vi "Variant Tools Test.vi"() -> ()   [LabVIEW 2017]
uses:
  c802287c-51b3-4527-ae67-bf64e1a5bd7d.vi
  fdbdbf5d-b64d-4e2e-bc22-f5c9394cad9c.vi
  <vilib>/addons/JSON API/JSON Value/Set from JSON string.vi
  Variant to JSON Text.vi
  JSON text to Variant.vi
  <vilib>/addons/JSON API/Variant JSON/Get as Variant.vi
  <vilib>/addons/JSON API/JSON Value/JSON Value.lvclass
  <vilib>/gmath/NI_Gmath.lvlib
  <vilib>/addons/JSON API/Get Polymorphic/JSON GetSet.lvlib
  <vilib>/addons/JSON API/Variant JSON/Variant JSON.lvlib
panel:
  in  "Pretty Print?":bool=TRUE
  out "x = y? 2":T1
  out "Cluster 2":T2={"A 6"=34, "T 1"="L", "A"=3, "<JSON>T 3"="", "T 4"="", "A 2"=1.23456, "T 5"="Test \"quote\",\nand newline.", "T 6"="sdfsdf", "A 3"=34, "Cluster 2"={"T 1"="SubCluster", "T 2"="Test \"quote\",\nand newline.", "A"=34, "T 3"="Test \"quote\",\nand newline.", "T 4"="Test \"quote\",\nand newline.", "A 2"=34, "T 5"="Test \"quote\",\nand newline.", "T 6"="Test \"quote\",\nand newline.", "A 3"=34}, "Array"=[1.23456, 1.23456, 1.23456, 1.23456, 1.23456, 1.23456, 1.23456, 1.23456, 1.23456, 1.23456, 1.23456, 1.23456, 2.23456]}
  in  "Old JSON":bool
  out "mean":dbl format="%.3p"
  out "length":i32
  out "Variant out":variant
  out "To Variant":dbl[](array[numeric]) format="%#_3p"
  in  "Cluster":T2={"A 6"=34, "T 1"="Line 1", "A"=34, "<JSON>T 3"="{\"T\":123}", "T 4"="sdfsdfdsfsdf", "A 2"=1.23456, "T 5"="Test \"quote\",\nand newline.", "T 6"="sdfsdf", "A 3"=34, "Cluster 2"={"T 1"="SubCluster", "T 2"="Test \"quote\",\nand newline.", "A"=34, "T 3"="Test \"quote\",\nand newline.", "T 4"="Test \"quote\",\nand newline.", "A 2"=34, "T 5"="Test \"quote\",\nand newline.", "T 6"="Test \"quote\",\nand newline.", "A 3"=34}, "Array"=[1.23456789, 1.23456789, 1.23456789, 1.23456789, 1.23456789, 1.23456789, 1.23456789, 1.23456789, 1.23456789, 1.23456789, 1.23456789, 1.23456789, 1.23456789, 1.23456789, 1.23456789, 1.23456789, 1.23456789, 1.23456789, 1.23456789, 1.23456789, 1.23456789, 1.23456789, 1.23456789, 1.23456789, 1.23456789, 1.23456789, 1.23456789, 1.23456789, 1.23456789, 1.23456789, 1.23456789, 1.23456789, 1.23456789, 1.23456789, 1.23456789, 1.23456789, 1.23456789, 1.23456789, 1.23456789, 1.23456789, 1.23456789, 1.23456789, 1.23456789, 1.23456789, 1.23456789, 1.23456789, 1.23456789, 1.23456789, 1.23456789, 1.23456789, 1.23456789, 1.23456789, 1.23456789, 1.23456789, 1.23456789, 1.23456789, 1.23456789, 1.23456789, 1.23456789, 1.23456789, 1.23456789, 1.23456789, 1.23456789, 1.23456789, 1.23456789, 1.23456789, 1.23456789, 1.23456789, 1.23456789, 1.23456789, 1.23456789, 1.23456789, 1.23456789, 1.23456789, 1.23456789, 1.23456789, 1.23456789, 1.23456789, 1.23456789, 1.23456789, 1.23456789, 1.23456789, 1.23456789, 1.23456789, 1.23456789, 1.23456789, 1.23456789, 1.23456789, 1.23456789, 1.23456789, 1.23456789, 1.23456789, 1.23456789, 1.23456789, 1.23456789, 1.23456789, 1.23456789, 1.23456789, 1.23456789, 1.23456789, 1.23456789, 1.23456789, 1.23456789, 1.23456789, 1.23456789, 1.23456789, 1.23456789, 1.23456789, 1.23456789, 1.23456789, 1.23456789, 1.23456789, 1.23456789, 1.23456789, 1.23456789, 1.23456789, 1.23456789, 1.23456789, 1.23456789, 1.23456789, 1.23456789, 1.23456789, 1.23456789, 1.23456789, 1.23456789, 1.23456789, 1.23456789, 1.23456789, 1.23456789, 1.23456789, 1.23456789, 1.23456789, 1.23456789, 1.23456789, 1.23456789, 1.23456789, 1.23456789, 1.23456789, 1.23456789, 1.23456789, 1.23456789, 1.23456789, 1.23456789, 1.23456789, 1.23456789, 1.23456789, 1.23456789, 1.23456789, 1.23456789, 1.23456789, 1.23456789, 1.23456789, 1.23456789, 1.23456789, 1.23456789, 1.23456789, 1.23456789, 1.23456789, 1.23456789, 1.23456789, 1.23456789, 1.23456789, 1.23456789, 1.23456789, 1.23456789, 1.23456789, 1.23456789, 1.23456789, 1.23456789, 1.23456789, 1.23456789, 1.23456789, 1.23456789, 1.23456789, 1.23456789, 1.23456789, 1.23456789, 1.23456789, 1.23456789, 1.23456789, 1.23456789, 1.23456789, 1.23456789, 1.23456789, 1.23456789, 1.23456789, 1.23456789, 1.23456789, 1.23456789, 1.23456789, 1.23456789, 1.23456789, 1.23456789, 1.23456789, 1.23456789, 1.23456789, 1.23456789, 1.23456789, 1.23456789, 1.23456789, 1.23456789, 1.23456789, 1.23456789, 1.23456789, 1.23456789, 1.23456789, 1.23456789, 1.23456789, 1.23456789, 1.23456789, 1.23456789, 1.23456789, 1.23456789, 1.23456789, 1.23456789, 1.23456789, 1.23456789, 1.23456789, 1.23456789, 1.23456789, 1.23456789, 1.23456789, 1.23456789, 1.23456789, 1.23456789, 1.23456789, 1.23456789, 1.23456789, 1.23456789, 1.23456789, 1.23456789, 1.23456789, 1.23456789, 1.23456789, 1.23456789, 1.23456789, 1.23456789, 1.23456789, 1.23456789, 1.23456789, 1.23456789, 1.23456789, 1.23456789, 1.23456789, 1.23456789, 1.23456789, 1.23456789, 1.23456789, 1.23456789, 1.23456789, 1.23456789, 1.23456789, 1.23456789, 1.23456789, 1.23456789, 1.23456789, 1.23456789, 1.23456789, 1.23456789, 1.23456789, 1.23456789, 1.23456789, 1.23456789, 1.23456789, 1.23456789, 1.23456789, 1.23456789, 1.23456789, 1.23456789, 1.23456789, 1.23456789, 1.23456789, 1.23456789, 1.23456789, 1.23456789, 1.23456789, 1.23456789, 1.23456789, 1.23456789, 1.23456789, 1.23456789, 1.23456789, 1.23456789, 1.23456789, 1.23456789, 1.23456789, 1.23456789, 1.23456789, 1.23456789, 1.23456789, 1.23456789, 1.23456789, 1.23456789, 1.23456789, 1.23456789, 1.23456789, 1.23456789, 1.23456789, 1.23456789, 1.23456789, 1.23456789, 1.23456789, 1.23456789, 1.23456789, 1.23456789, 1.23456789, 1.23456789, 1.23456789, 1.23456789, 1.23456789, 1.23456789, 1.23456789, 1.23456789, 1.23456789, 1.23456789, 1.23456789, 1.23456789, 1.23456789, 1.23456789, 1.23456789, 1.23456789, 1.23456789, 1.23456789, 1.23456789, 1.23456789, 1.23456789, 1.23456789, 1.23456789, 1.23456789, 1.23456789, 1.23456789, 1.23456789, 1.23456789, 1.23456789, 1.23456789, 1.23456789, 1.23456789, 1.23456789, 1.23456789, 1.23456789, 1.23456789, 1.23456789, 1.23456789, 1.23456789, 1.23456789, 1.23456789, 1.23456789, 1.23456789, 1.23456789, 1.23456789, 1.23456789, 1.23456789, 1.23456789, 1.23456789, 1.23456789, 1.23456789, 1.23456789, 1.23456789, 1.23456789, 1.23456789, 1.23456789, 1.23456789, 1.23456789, 1.23456789, 1.23456789, 1.23456789, 1.23456789, 1.23456789, 1.23456789, 1.23456789, 1.23456789, 1.23456789, 1.23456789, 1.23456789, 1.23456789, 1.23456789, 1.23456789, 1.23456789, 1.23456789, 1.23456789, 1.23456789, 1.23456789, 1.23456789, 1.23456789, 1.23456789, 1.23456789, 1.23456789, 1.23456789, 1.23456789, 1.23456789, 1.23456789, 1.23456789, 1.23456789, 1.23456789, 1.23456789, 1.23456789, 1.23456789, 1.23456789, 1.23456789, 1.23456789, 1.23456789, 1.23456789, 1.23456789, 1.23456789, 1.23456789, 1.23456789, 1.23456789, 1.23456789, 1.23456789, 1.23456789, 1.23456789, 1.23456789, 1.23456789, 1.23456789, 1.23456789, 1.23456789, 1.23456789, 1.23456789, 1.23456789, 1.23456789, 1.23456789, 1.23456789, 1.23456789, 1.23456789, 1.23456789, 1.23456789, 1.23456789, 1.23456789, 1.23456789, 1.23456789, 1.23456789, 1.23456789, 1.23456789, 1.23456789, 1.23456789, 1.23456789, 1.23456789, 1.23456789, 1.23456789, 1.23456789, 1.23456789, 1.23456789, 1.23456789, 1.23456789, 1.23456789, 1.23456789, 1.23456789, 1.23456789, 1.23456789, 1.23456789, 1.23456789, 1.23456789, 1.23456789, 1.23456789, 1.23456789, 1.23456789, 1.23456789, 1.23456789, 1.23456789, 1.23456789, 1.23456789, 1.23456789, 1.23456789, 1.23456789, 1.23456789, 1.23456789, 1.23456789, 1.23456789, 1.23456789, 1.23456789, 1.23456789, 1.23456789, 1.23456789, 1.23456789, 1.23456789, 1.23456789, 1.23456789, 1.23456789, 1.23456789, 1.23456789, 1.23456789, 1.23456789, 1.23456789, 1.23456789, 1.23456789, 1.23456789, 1.23456789, 1.23456789, 1.23456789, 1.23456789, 1.23456789, 1.23456789, 1.23456789, 1.23456789, 1.23456789, 1.23456789, 1.23456789, 1.23456789, 1.23456789, 1.23456789, 1.23456789, 1.23456789, 1.23456789, 1.23456789, 1.23456789, 1.23456789, 1.23456789, 1.23456789, 1.23456789, 1.23456789, 1.23456789, 1.23456789, 1.23456789, 1.23456789, 1.23456789, 1.23456789, 1.23456789, 1.23456789, 1.23456789, 1.23456789, 1.23456789, 1.23456789, 1.23456789, 1.23456789, 1.23456789, 1.23456789, 1.23456789, 1.23456789, 1.23456789, 1.23456789, 1.23456789, 1.23456789, 1.23456789, 1.23456789, 1.23456789, 1.23456789, 1.23456789, 1.23456789, 1.23456789, 1.23456789, 1.23456789, 1.23456789, 1.23456789, 1.23456789, 1.23456789, 1.23456789, 1.23456789, 1.23456789, 1.23456789, 1.23456789, 1.23456789, 1.23456789, 1.23456789, 1.23456789, 1.23456789, 1.23456789, 1.23456789, 1.23456789, 1.23456789, 1.23456789, 1.23456789, 1.23456789, 1.23456789, 1.23456789, 1.23456789, 1.23456789, 1.23456789, 1.23456789, 1.23456789, 1.23456789, 1.23456789, 1.23456789, 1.23456789, 1.23456789, 1.23456789, 1.23456789, 1.23456789, 1.23456789, 1.23456789, 1.23456789, 1.23456789, 1.23456789, 1.23456789, 1.23456789, 1.23456789, 1.23456789, 1.23456789, 1.23456789, 1.23456789, 1.23456789, 1.23456789, 1.23456789, 1.23456789, 1.23456789, 1.23456789, 1.23456789, 1.23456789, 1.23456789, 1.23456789, 1.23456789, 1.23456789, 1.23456789, 1.23456789, 1.23456789, 1.23456789, 1.23456789, 1.23456789, 1.23456789, 1.23456789, 1.23456789, 1.23456789, 1.23456789, 1.23456789, 1.23456789, 1.23456789, 1.23456789, 1.23456789, 1.23456789, 1.23456789, 1.23456789, 1.23456789, 1.23456789, 1.23456789, 1.23456789, 1.23456789, 1.23456789, 1.23456789, 1.23456789, 1.23456789, 1.23456789, 1.23456789, 1.23456789, 1.23456789, 1.23456789, 1.23456789, 1.23456789, 1.23456789, 1.23456789, 1.23456789, 1.23456789, 1.23456789, 1.23456789, 1.23456789, 1.23456789, 1.23456789, 1.23456789, 1.23456789, 1.23456789, 1.23456789, 1.23456789, 1.23456789, 1.23456789, 1.23456789, 1.23456789, 1.23456789, 1.23456789, 1.23456789, 1.23456789, 1.23456789, 1.23456789, 1.23456789, 1.23456789, 1.23456789, 1.23456789, 1.23456789, 1.23456789, 1.23456789, 1.23456789, 1.23456789, 1.23456789, 1.23456789, 1.23456789, 1.23456789, 1.23456789, 1.23456789, 1.23456789, 1.23456789, 1.23456789, 1.23456789, 1.23456789, 1.23456789, 1.23456789, 1.23456789, 1.23456789, 1.23456789, 1.23456789, 1.23456789, 1.23456789, 1.23456789, 1.23456789, 1.23456789, 1.23456789, 1.23456789, 1.23456789, 1.23456789, 1.23456789, 1.23456789, 1.23456789, 1.23456789, 1.23456789, 1.23456789, 1.23456789, 1.23456789, 1.23456789, 1.23456789, 1.23456789, 1.23456789, 1.23456789, 1.23456789, 1.23456789, 1.23456789, 1.23456789, 1.23456789, 1.23456789, 1.23456789, 1.23456789, 1.23456789, 1.23456789, 1.23456789, 1.23456789, 1.23456789, 1.23456789, 1.23456789, 1.23456789, 1.23456789, 1.23456789, 1.23456789, 1.23456789, 1.23456789, 1.23456789, 1.23456789, 1.23456789, 1.23456789, 1.23456789, 1.23456789, 1.23456789, 1.23456789, 1.23456789, 1.23456789, 1.23456789, 1.23456789, 1.23456789, 1.23456789, 1.23456789, 1.23456789, 1.23456789, 1.23456789, 1.23456789, 1.23456789, 1.23456789, 1.23456789, 1.23456789, 1.23456789, 1.23456789, 1.23456789, 1.23456789, 1.23456789, 1.23456789, 1.23456789, 1.23456789, 1.23456789, 1.23456789, 1.23456789, 1.23456789, 1.23456789, 1.23456789, 1.23456789, 1.23456789, 1.23456789, 1.23456789, 1.23456789, 1.23456789, 1.23456789, 1.23456789, 1.23456789, 1.23456789, 1.23456789, 1.23456789, 1.23456789, 1.23456789, 1.23456789, 1.23456789, 1.23456789, 1.23456789, 1.23456789, 1.23456789, 1.23456789, 1.23456789, 1.23456789, 1.23456789, 1.23456789, 1.23456789, 1.23456789, 1.23456789, 1.23456789, 1.23456789, 1.23456789, 1.23456789, 1.23456789, 1.23456789, 1.23456789, 1.23456789, 1.23456789, 1.23456789, 1.23456789, 1.23456789, 1.23456789, 1.23456789, 1.23456789, 1.23456789, 1.23456789, 1.23456789, 1.23456789, 1.23456789, 1.23456789, 1.23456789, 1.23456789, 1.23456789, 1.23456789, 1.23456789, 1.23456789, 1.23456789, 1.23456789, 1.23456789, 1.23456789, 1.23456789, 1.23456789, 1.23456789, 1.23456789, 1.23456789, 1.23456789, 1.23456789, 1.23456789, 1.23456789, 1.23456789, 1.23456789, 1.23456789, 1.23456789, 1.23456789, 1.23456789, 1.23456789, 1.23456789, 1.23456789, 1.23456789, 1.23456789, 1.23456789, 1.23456789, 1.23456789, 1.23456789, 1.23456789, 1.23456789, 1.23456789, 1.23456789, 1.23456789, 1.23456789, 1.23456789, 1.23456789, 1.23456789, 1.23456789, 1.23456789, 1.23456789, 1.23456789, 1.23456789, 1.23456789, 1.23456789, 1.23456789, 1.23456789, 1.23456789, 1.23456789, 1.23456789, 1.23456789, 1.23456789, 1.23456789, 1.23456789, 1.23456789, 1.23456789, 1.23456789, 1.23456789, 1.23456789, 1.23456789, 1.23456789, 1.23456789, 1.23456789, 1.23456789, 1.23456789, 1.23456789, 1.23456789, 1.23456789, 1.23456789, 1.23456789, 1.23456789, 1.23456789, 1.23456789, 1.23456789, 1.23456789, 1.23456789, 1.23456789, 1.23456789, 1.23456789, 1.23456789, 1.23456789, 1.23456789, 1.23456789, 1.23456789, 1.23456789, 1.23456789, 1.23456789, 1.23456789, 1.23456789, 1.23456789, 1.23456789, 1.23456789, 1.23456789, 1.23456789, 1.23456789, 1.23456789, 1.23456789, 1.23456789, 1.23456789, 1.23456789, 1.23456789, 1.23456789, 1.23456789, 1.23456789, 1.23456789, 1.23456789, 1.23456789, 1.23456789, 1.23456789, 1.23456789, 1.23456789, 1.23456789, 1.23456789, 1.23456789, 1.23456789, 1.23456789, 1.23456789, 1.23456789, 1.23456789, 1.23456789, 1.23456789, 1.23456789, 1.23456789, 1.23456789, 1.23456789, 1.23456789, 1.23456789, 1.23456789, 1.23456789, 1.23456789, 1.23456789, 1.23456789, 1.23456789, 1.23456789, 1.23456789, 1.23456789, 1.23456789, 1.23456789, 1.23456789, 1.23456789, 1.23456789, 1.23456789, 1.23456789, 1.23456789, 1.23456789, 1.23456789, 1.23456789, 1.23456789, 1.23456789, 1.23456789, 1.23456789, 1.23456789, 1.23456789, 1.23456789, 1.23456789, 1.23456789, 1.23456789, 1.23456789, 1.23456789, 1.23456789, 1.23456789, 1.23456789, 1.23456789, 1.23456789, 1.23456789, 1.23456789, 1.23456789, 1.23456789, 1.23456789, 1.23456789, 1.23456789, 1.23456789, 1.23456789, 1.23456789, 1.23456789, 1.23456789, 1.23456789, 1.23456789, 1.23456789, 1.23456789, 2.23456789]}
  out "<JSON>":string
  out "error out":errorcluster
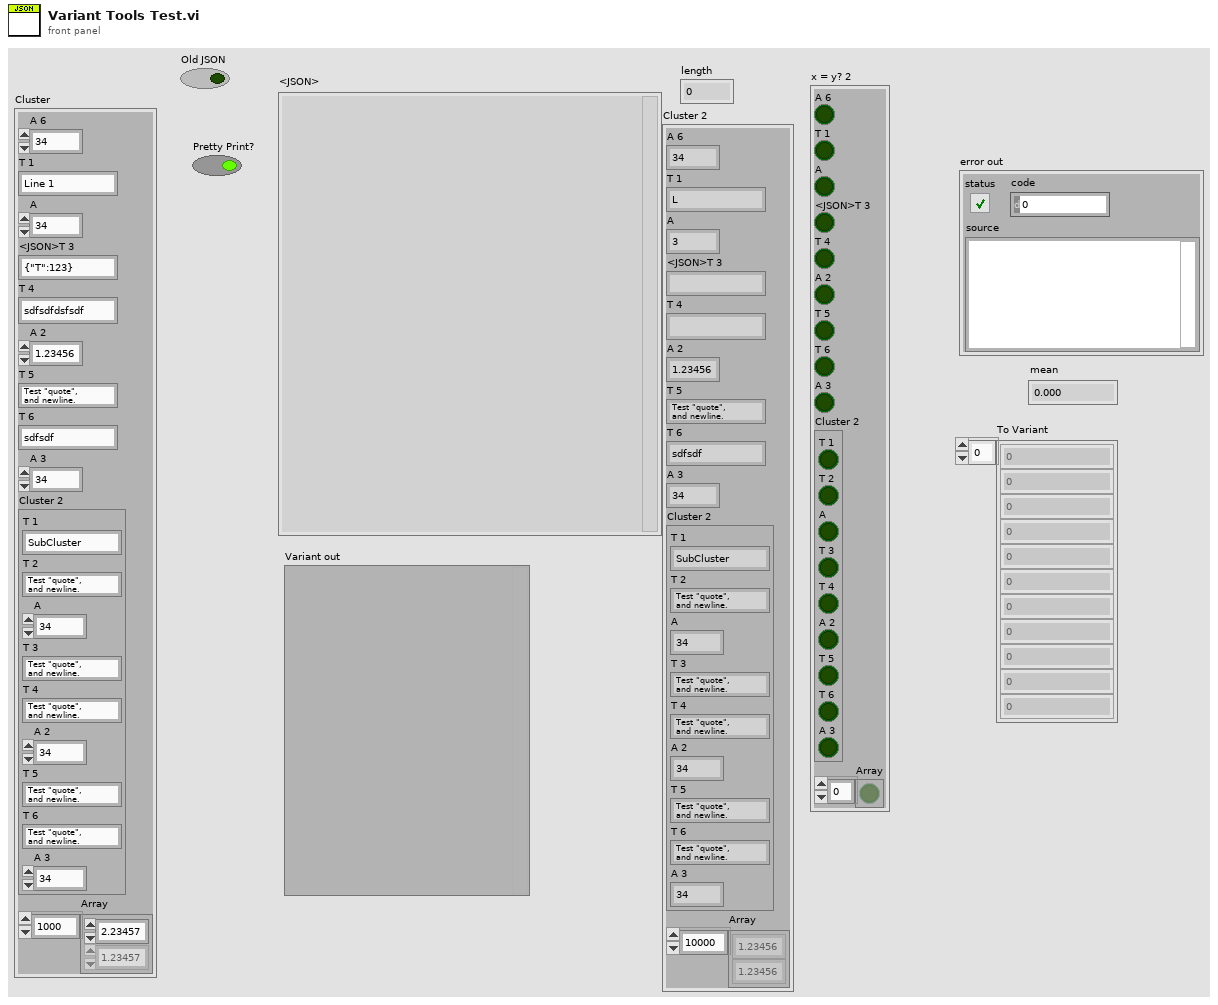
[diagram p1: front panel]
types:
  T1 = cluster{"A 6":bool, "T 1":bool, "A":bool, "<JSON>T 3":bool, "T 4":bool, "A 2":bool, "T 5":bool, "T 6":bool, "A 3":bool, "Cluster 2":cluster{"T 1":bool, "T 2":bool, "A":bool, "T 3":bool, "T 4":bool, "A 2":bool, "T 5":bool, "T 6":bool, "A 3":bool}, "Array":bool[]}
  T2 = cluster{"A 6":i32, "T 1":string, "A":i32, "<JSON>T 3":string, "T 4":string, "A 2":dbl, "T 5":string, "T 6":string, "A 3":i32, "Cluster 2":cluster{"T 1":string, "T 2":string, "A":i32, "T 3":string, "T 4":string, "A 2":i32, "T 5":string, "T 6":string, "A 3":i32}, "Array":dbl[]}
  T3 = enum16{"arithmetic", "geometric", "harmonic", "trimmed", "median"}
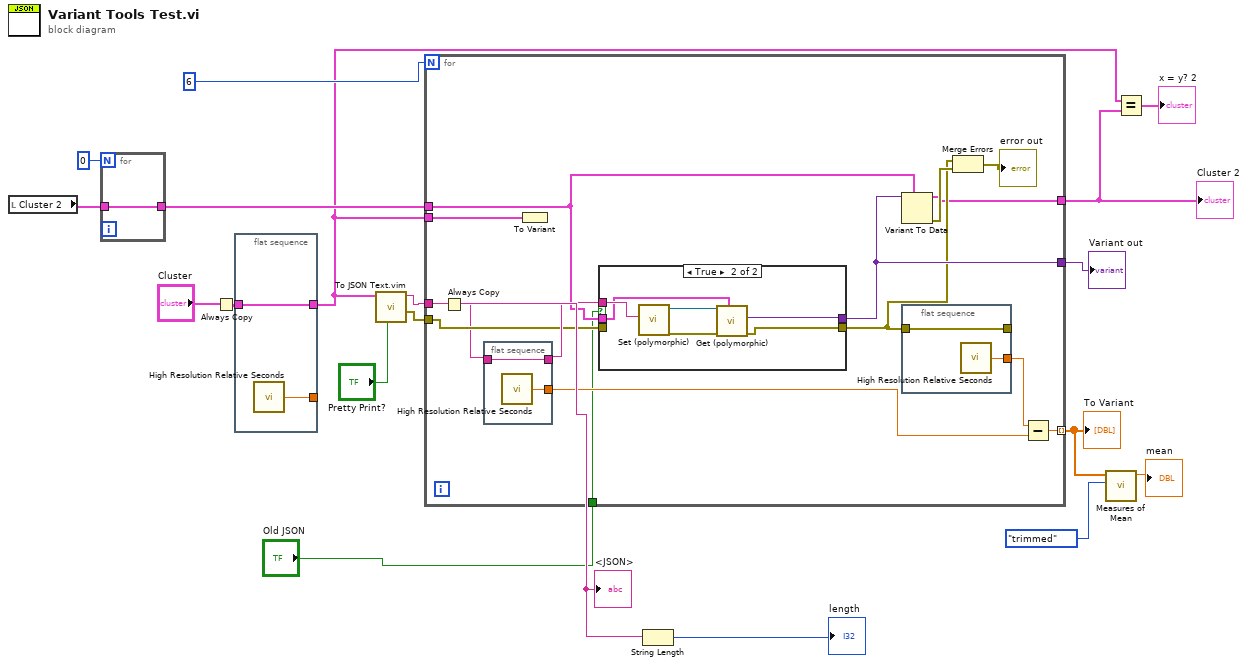
[diagram p0: block diagram]
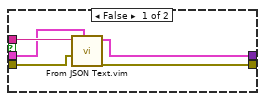
[diagram p2: hidden frame]
diagram:
  n1 = local read "Cluster 2"() -> (w15:T2)
  n2 = for {
    N: 0 -> [_]
    tunnel: [w19] -> w16
    tunnel: w15 -> [w19]
  }
  n3 = Always Copy(1:"Cluster") -> (0:w11:T2)
  n4 = flat-sequence {
    tunnel: w11 -> [w20]
    tunnel: [w21] -> _
    tunnel: [w20] -> w1
    frame #0 {
      n5 = call <vilib>:"High Resolution Relative Seconds.vi"() -> ("relative seconds"=w21:dbl)
    }
  }
  n6 = call "To JSON Text.vim"("Pretty Print?"="Pretty Print?", "Variant"=w1) -> ("error out"=w2:errorcluster, "<JSON>"=w9:string)  [unwired: 8 in]
  "<JSON>" <- w9
  n7 = for {
    N: 6 -> [_]
    tunnel: [w36] -> w7 mode=indexing
    tunnel: w16 -> [w35]
    tunnel: w9 -> [w27]
    tunnel: [w22] -> w4
    tunnel: [w34] -> w13
    tunnel: w1 -> [w31]
    tunnel: w2 -> [w25]
    tunnel: "Old JSON" -> [w23]
    n8 = Always Copy(1:w27) -> (0:w24:string)
    n9 = flat-sequence {
      tunnel: [w49] -> w26
      tunnel: w24 -> [w49]
      tunnel: [w48] -> w30
      frame #0 {
        n10 = call <vilib>:"High Resolution Relative Seconds.vi"() -> ("relative seconds"=w48:dbl)
      }
    }
    n11 = To Variant(anything=w31) -> ()  [unwired: 1 out]
    n12 = case shown="True" w23 {
      tunnel: w35 -> [w40 w46]
      tunnel: [w38 w44] -> w34
      tunnel: [w37 w43] -> w28
      tunnel: w26 -> [w41 w47]
      tunnel: w25 -> [w39 _]
      frame False {
        n13 = call "From JSON Text.vim"("Data Type and Default Value"=w40, "error in (no error)"=w39, "JSON"=w41) -> ("error out"=w37:errorcluster, "Variant out"=w38:T2)  [unwired: 7 in]
      }
      frame True {
        n14 = call-poly <vilib>:"Set (polymorphic).vi"("JSON stream"=w47) -> ("error out"=w42:errorcluster, "JSON Value out"=w45:refnum<class "JSON Value.lvclass">)  [unwired: 8 in, 1 out]
        n15 = call-poly <vilib>:"Get (polymorphic).vi"("Variant (Data Type)"=w46, "error in (no error)"=w42, "JSON in"=w45) -> ("error out"=w43:errorcluster, "Variant out"=w44:variant)  [unwired: 6 in, 1 out]
      }
    }
    n16 = Variant To Data(type=w35, Variant=w34) -> (data=w22:T2, error out=w33:errorcluster)  [unwired: 1 in]
    n17 = flat-sequence {
      tunnel: [w51] -> _
      tunnel: w28 -> [w51]
      tunnel: [w50] -> w32
      frame #0 {
        n18 = call <vilib>:"High Resolution Relative Seconds.vi"() -> ("relative seconds"=w50:dbl)
      }
    }
    n19 = Merge Errors(w28, w33) -> (→"error out":errorcluster)
    n20 = Subtract(x=w32, y=w30) -> (x-y=w36:dbl)
  }
  "To Variant" <- w7
  "Variant out" <- w13
  "Cluster 2" <- w4
  n21 = String Length(string=w9) -> (length=→"length":i32)
  n22 = call <vilib>:"Measures of Mean.vi"("type"=T3."trimmed", "x array"=w7) -> ("mean value"=→"mean":dbl)  [unwired: 8 in, 1 out]
  n23 = Equal?(x=w1, y=w4) -> (x = y?=→"x = y? 2":T1)
